vi "input_32_bit_channel_producer.vi"(7 "Index":i32, 8 "error in (no error)":errorcluster, 9 "aData Out":dbl[][](array[numeric]), 10 "DirQ":refnum<queue>) -> (0 "error out":errorcluster)   [LabVIEW 2025, in "LabJackEKG.lvlib"]
uses:
  LabJackEKG.lvlib
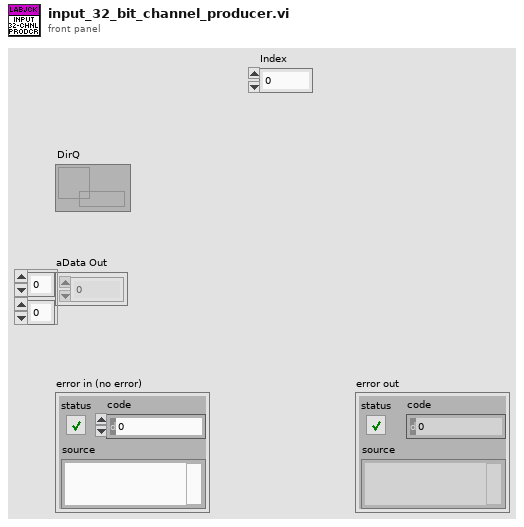
[diagram p1: front panel]
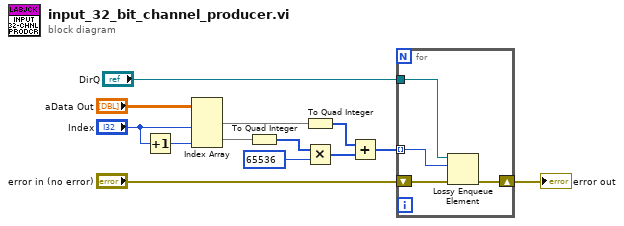
[diagram p0: block diagram]
diagram:
  n1 = Increment(x="Index") -> (x+1=w2:i32)
  n2 = Index Array(array="aData Out", index (col) #1="Index", index (col) #2=w2) -> (element #1=w8:dbl[], element #2=w7:dbl[])  [unwired: 2 in]
  n3 = To Quad Integer(1:w7) -> (0:w9:i64[])
  n4 = To Quad Integer(1:w8) -> (0:w4:i64[])
  n5 = Multiply(x=w9, y=i64 65536 ("x")) -> (x*y=w5:i64[])
  n6 = Add(x=w4, y=w5) -> (x+y=w6:i64[])
  n7 = for {
    tunnel: "DirQ" -> [w17]
    shift-right: [w16] -> w13
    shift-left: "error in (no error)" -> [w15]
    tunnel: w6 -> [w14] mode=indexing
    n8 = Lossy Enqueue Element(queue=w17, element=w14, error in (no error)=w15) -> (error out=w16:errorcluster)  [unwired: 3 out]
  }
  "error out" <- w13
